vi "cRIO_FPGA_COMMUNICATION Read and Sort Data of all Stations.vi"(8 "error in (no error)":errorcluster caption="Fehler (Eingang, kein Fehler)", 11 "FPGA-VI-Referenz (Ausgang)":refnum<k20>) -> (0 "error out":errorcluster, 1 "Zählerwerte (super schneller Counter)":u16[](array[numeric]), 3 "Band & Stationsdaten":u16[](array[numeric]))   [LabVIEW 2013, in "cRIO_FPGA_COMMUNICATION.lvlib"]
uses:
  cRIO_FPGA_COMMUNICATION.lvlib
  <vilib>/Utility/error.llb/Error Cluster From Error Code.vi
  <vilib>/rvi/errors/niLvFpgaAdjustHostInterfaceError.vi
  <vilib>/rvi/interface/common/niFpgaWaitOnOcc.vi
  <vilib>/rvi/interface/nirviReadWriteControl/nirviReadWriteControl.xnode
  FPGA Bitfiles/Test_FPGATarget_CScRIOPBFPGADP-M_4E0AD52E.lvbitx
  <vilib>/rvi/interface/nirviMethod/nirviMethod.xnode
  <vilib>/rvi/errors/niLvFpgaMergeErrorWithErrorCode.vi
  <vilib>/FPGAPlugInAG/cRIO-9114/niLvFpga_ReadFifo_cRIO-9114.vi
  NiFpgaLv.dll
panel:
  out "Zeit seit letztem Aufruf [us]":u32
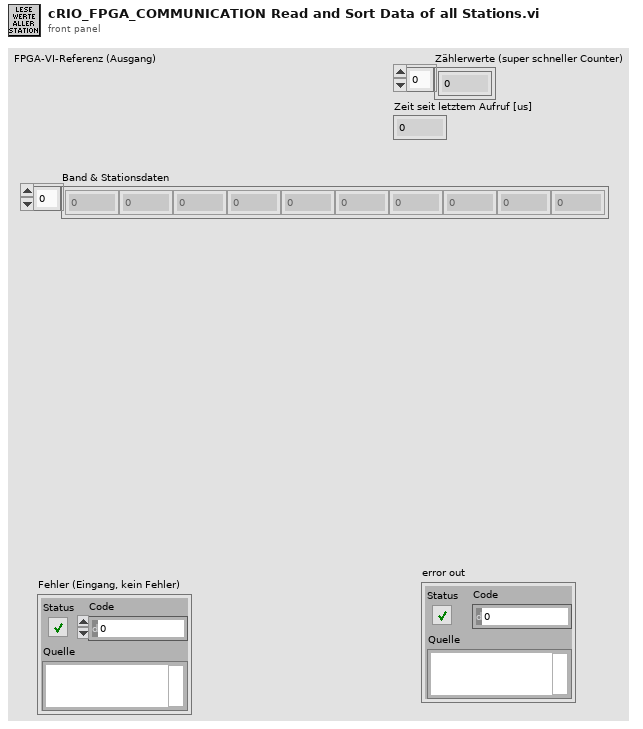
[diagram p1: front panel]
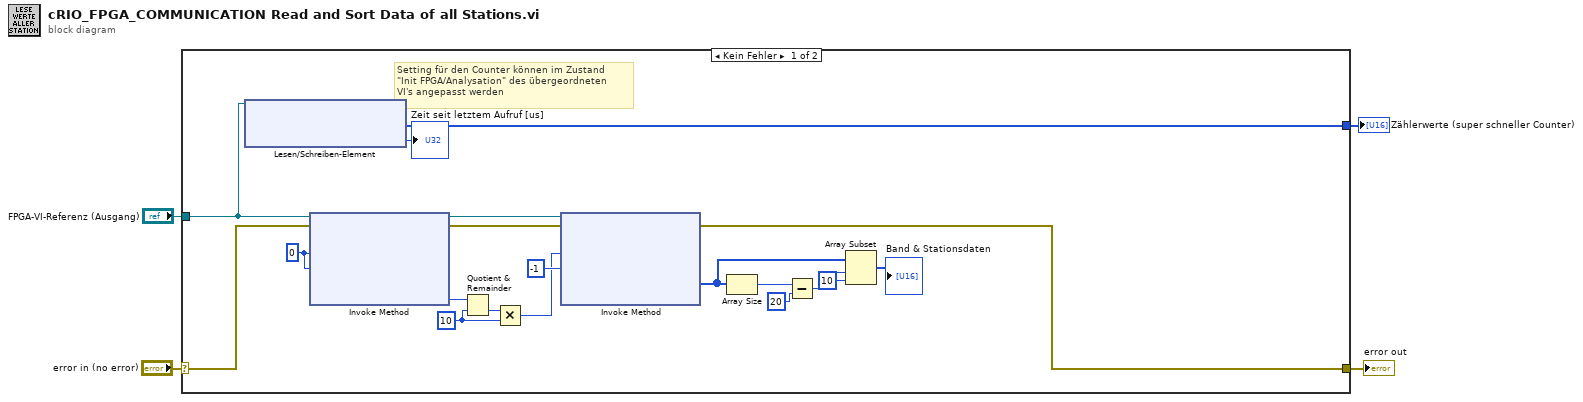
[diagram p0: block diagram]
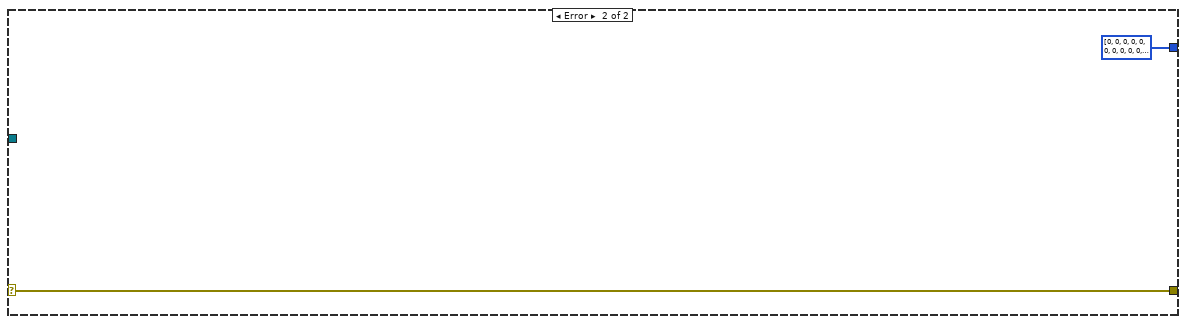
[diagram p2: hidden frame]
diagram:
  n1 = case shown="Kein Fehler" "error in (no error)" {
    selector: "error in (no error)" -> [w23 w25]
    tunnel: "FPGA-VI-Referenz (Ausgang)" -> [w20 _]
    tunnel: [w22 w25] -> w4
    tunnel: [w21 u16[] [0, 0, 0, 0, 0, 0, 0, 0, 0, 0, 0, 0, 0, 0, 0, 0, 0, 0, 0, 0, 0, 0, 0, 0, 0, 0, 0, 0, 0, 0] ("Zählerwerte")] -> w1
    frame No Error {
      w19 = u8 10
      w17 = u32 0 ("Anzahl der Elemente")
      # "Setting für den Counter können im Zustand\n\"Init FPGA/Analysation\" des übergeordneten\nVI's angepasst werden"
      n2 = xnode "Lesen/Schreiben-Element"("FPGA-VI-Referenz (Eingang)"=w20) -> ("Zählerwerte"=w21:u16[], "Zeit seit letztem Aufruf [us]"=→"Zeit seit letztem Aufruf [us]":u32)  [unwired: 1 in, 2 out]
      n3 = xnode "Invoke Method"("FPGA-VI-Referenz (Eingang)"=w20, "Fehler (Eingang)"=w23, "Anzahl der Elemente"=w17, "Timeout (ms)"=w17) -> ("FPGA-VI-Referenz (Ausgang)"=w13:refnum<k20>, "Fehler (Ausgang)"=w14:errorcluster, "Verbleibende Elemente"=w15:u32)  [unwired: 1 out]
      n4 = Quotient & Remainder(x=w15, y=w19) -> (floor(x/y)=w16:u32)  [unwired: 1 out]
      n5 = Multiply(x=w16, y=w19) -> (x*y=w12:u32)
      n6 = xnode "Invoke Method"("FPGA-VI-Referenz (Eingang)"=w13, "Fehler (Eingang)"=w14, "Anzahl der Elemente"=w12, "Timeout (ms)"=-1) -> ("Fehler (Ausgang)"=w22:errorcluster, "Daten"=w11:u16[])  [unwired: 2 out]
      n7 = Array Size(array=w11) -> (size(s)=w10:i32)
      n8 = Subtract(x=w10, y=20) -> (x-y=w8:i32)
      n9 = Array Subset(array=w11, index=w8, length=10 ("Länge")) -> (→"Band & Stationsdaten":u16[])
    }
    frame Error {
    }
  }
  "error out" <- w4
  "Zählerwerte (super schneller Counter)" <- w1
